vi "GUI_148_AmplifierCamsV2.vi"() -> ()   [LabVIEW 2013]
uses:
  shared programs/GUI_Template/GUI_master/tcp_new_data_event.ctl
  shared programs/GUI_Template/GUI_master/tcp new data cluster.ctl
  <userlib>/_OpenG.lib/array/array.llb/Filter 1D Array with Scalar (String)__ogtk.vi
panel:
  in  "TargetSize.Y::7":dbl=45.0 caption="y" min=2.0 max=3000.0 format="%#_6f"
  in  "TargetSize.X::7":dbl=47.0 caption="x" min=2.0 max=3000.0 format="%#_6f"
  in  "TargetSize.Y::6":dbl=45.0 caption="y" min=2.0 max=3000.0 format="%#_6f"
  in  "TargetSize.X::6":dbl=47.0 caption="x" min=2.0 max=3000.0 format="%#_6f"
  in  "TargetSize.Y::5":dbl=45.0 caption="y" min=2.0 max=3000.0 format="%#_6f"
  in  "TargetSize.X::5":dbl=47.0 caption="x" min=2.0 max=3000.0 format="%#_6f"
  in  "TargetSize.Y::4":dbl=45.0 caption="y" min=2.0 max=3000.0 format="%#_6f"
  in  "TargetSize.X::4":dbl=47.0 caption="x" min=2.0 max=3000.0 format="%#_6f"
  in  "TargetSize.Y::3":dbl=163.0 caption="y" min=2.0 max=3000.0 format="%#_6f"
  in  "TargetSize.X::3":dbl=152.0 caption="x" min=2.0 max=3000.0 format="%#_6f"
  in  "TargetSize.Y::2":dbl=74.0 caption="y" min=2.0 max=3000.0 format="%#_6f"
  in  "TargetSize.X::2":dbl=75.0 caption="x" min=2.0 max=3000.0 format="%#_6f"
  in  "active cams":string
  out "CCDs":string[](array[string])
  out "Cameras":T1
  in  "Target.Y::7":dbl=45.0 caption="y" min=0.0 max=2000.0 format="%#_6f"
  in  "Target.X::7":dbl=47.0 caption="x" min=0.0 max=2000.0 format="%#_6f"
  in  "Target.Y::6":dbl=45.0 caption="y" min=0.0 max=2000.0 format="%#_6f"
  in  "Target.X::6":dbl=47.0 caption="x" min=0.0 max=2000.0 format="%#_6f"
  in  "Target.Y::5":dbl=45.0 caption="y" min=0.0 max=2000.0 format="%#_6f"
  in  "Target.X::5":dbl=47.0 caption="x" min=0.0 max=2000.0 format="%#_6f"
  in  "Target.Y::4":dbl=45.0 caption="y" min=0.0 max=2000.0 format="%#_6f"
  in  "Target.X::4":dbl=47.0 caption="x" min=0.0 max=2000.0 format="%#_6f"
  in  "Target.Y::3":dbl=163.0 caption="y" min=0.0 max=2000.0 format="%#_6f"
  in  "Target.X::3":dbl=152.0 caption="x" min=0.0 max=2000.0 format="%#_6f"
  in  "Target.Y::2":dbl=74.0 caption="y" min=0.0 max=2000.0 format="%#_6f"
  in  "Target.X::2":dbl=75.0 caption="x" min=0.0 max=2000.0 format="%#_6f"
  out "error out":errorcluster
  out "image::7":T2(plugin-control) caption="U_Amp3GaiaBay"
  in  "triggerdelay::7":dbl=0.001 caption="triggerdelay" min=0.0 max=50000.0 format="%_4p"
  in  "triggerdelay::6":dbl=0.001 caption="triggerdelay" min=20.0 max=50000.0 format="%_4p"
  in  "triggerdelay::5":dbl=0.001 caption="triggerdelay" min=10.0 max=50000.0 format="%_4p"
  in  "triggerdelay::4":dbl=0.001 caption="triggerdelay" min=0.0 max=50000.0 format="%_4p"
  in  "triggerdelay::3":dbl=0.001 caption="triggerdelay" min=20.0 max=50000.0 format="%_4p"
  in  "triggerdelay::2":dbl=0.001 caption="triggerdelay" min=0.0 max=50000.0 format="%_4p"
  in  "trigger::7":bool caption="Trigger"
  in  "centroidy::7":dbl=0.001 caption="centroid y" min=0.0 max=0.0 format="%_4f"
  in  "centroidx::7":dbl=0.001 caption="centroid x" min=0.0 max=0.0 format="%_4f"
  in  "exposure::7":dbl=0.001 caption="exposure" min=0.0001 max=1.0 format="%_4p"
  in  "GUIdevice 7":string="U_GAIACam"
  in  "trigger::6":bool caption="Trigger"
  in  "centroidy::6":dbl=0.001 caption="centroid y" min=0.0 max=0.0 format="%_4f"
  in  "centroidx::6":dbl=0.001 caption="centroid x" min=0.0 max=0.0 format="%_4f"
  in  "exposure::6":dbl=0.001 caption="exposure" min=0.0001 max=1.0 format="%_4p"
  out "image::6":T2(plugin-control) caption="U_Amp3GaiaBay"
  in  "GUIdevice 6":string="U_Amp3GaiaBay"
  in  "trigger::5":bool caption="Trigger"
  in  "centroidy::5":dbl=0.001 caption="centroid y" min=0.0 max=0.0 format="%_4f"
  in  "centroidx::5":dbl=0.001 caption="centroid x" min=0.0 max=0.0 format="%_4f"
  in  "exposure::5":dbl=0.001 caption="exposure" min=0.0001 max=1.0 format="%_4p"
  out "image::5":T2(plugin-control) caption="U_Amp2GaiaBay"
  in  "GUIdevice 5":string="U_Amp2GaiaBay"
  in  "trigger::4":bool caption="Trigger"
  in  "centroidy::4":dbl=0.001 caption="centroid y" min=0.0 max=0.0 format="%_4f"
  in  "centroidx::4":dbl=0.001 caption="centroid x" min=0.0 max=0.0 format="%_4f"
  in  "exposure::4":dbl=0.001 caption="exposure" min=1e-06 max=1.0 format="%_4p"
  out "image::4":T2(plugin-control) caption="U_IRMobileImager"
  in  "GUIdevice 4":string="U_IRMobileImager"
  in  "trigger::3":bool caption="Trigger"
  in  "centroidy::3":dbl=0.001 caption="centroid y" min=0.0 max=0.0 format="%_4f"
  in  "centroidx::3":dbl=0.001 caption="centroid x" min=0.0 max=0.0 format="%_4f"
  in  "exposure::3":dbl=0.001 caption="exposure" min=0.0001 max=1.0 format="%_4p"
  out "image::3":T2(plugin-control) caption="Amp3_IR_Input"
  in  "GUIdevice 3":string="U_Amp3_IR_Input"
  in  "trigger::2":bool caption="Trigger"
  in  "centroidy::2":dbl=0.001 caption="centroid y" min=0.0 max=0.0 format="%_4f"
  in  "centroidx::2":dbl=0.001 caption="centroid x" min=0.0 max=0.0 format="%_4f"
  in  "exposure::2":dbl=0.001 caption="exposure" min=0.0001 max=1.0 format="%_4p"
  out "image::2":T2(plugin-control) caption="Amp2_IR_input"
  in  "GUIdevice 2":string="U_Amp2_IR_input"
  out "tcp data event":T3
  in  "Refresh Button":bool caption="Update Crosshairs"
  in  "Select device":string(combo)="FrogHPD"
  in  "stop":bool
  in  "GUIdevice 1":string="HPD_CCD"
  # "XHair location"
  # "XHair size"
  # "XHair location"
  # "XHair size"
  # "XHair location"
  # "XHair size"
  # "XHair location"
  # "XHair size"
  # "XHair location"
  # "XHair size"
  # "XHair location"
  # "XHair size"
  # "XHair location"
  # "XHair size"
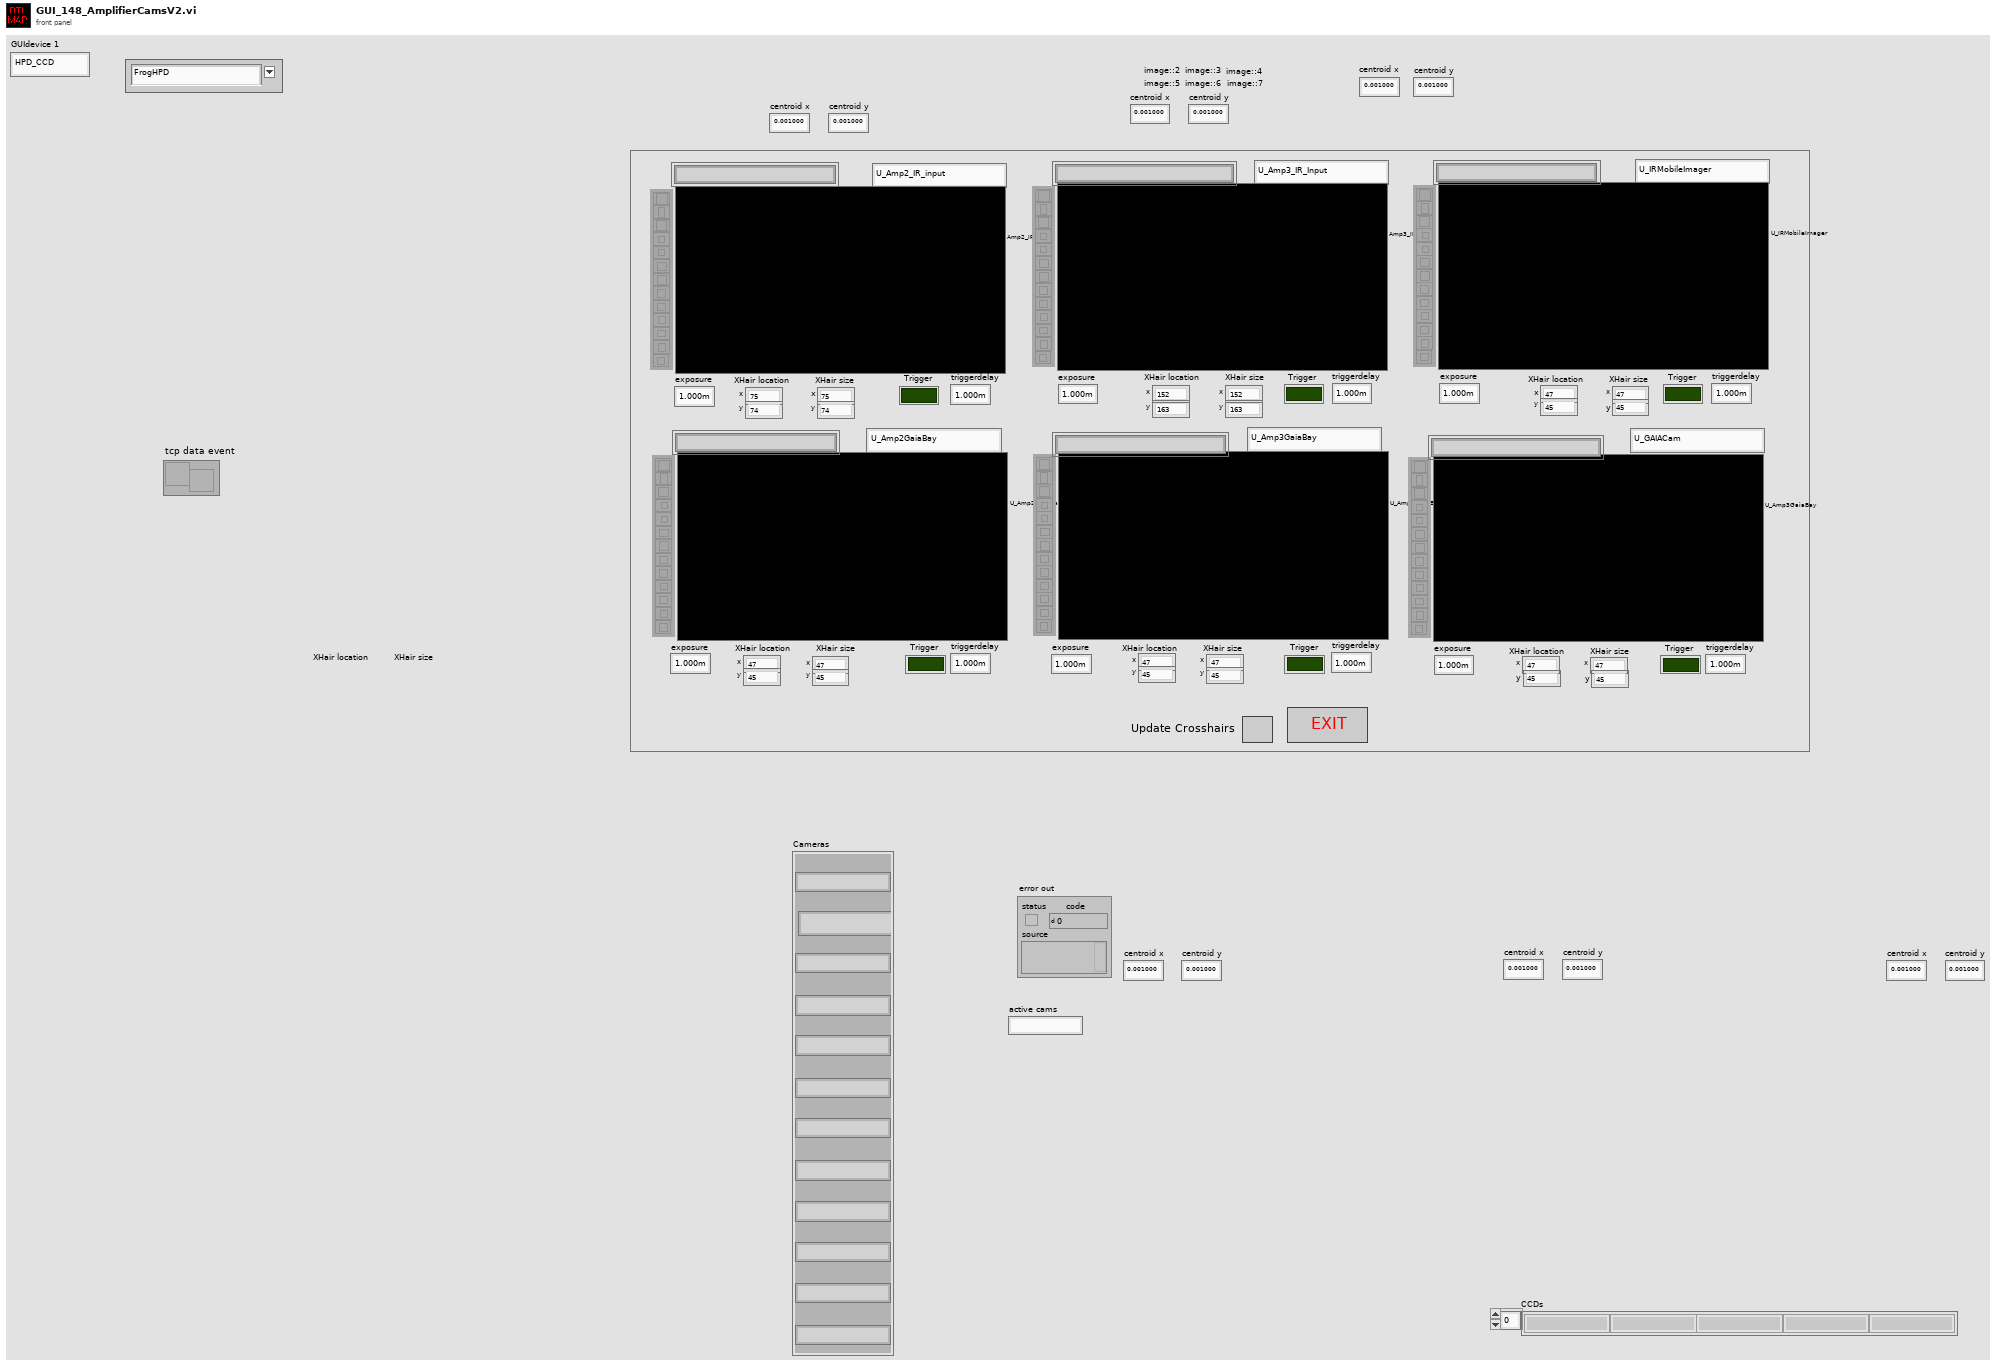
[diagram p1: front panel]
types:
  T1 = cluster{"[0]":string, "[1]":string, "[2]":string, "[3]":string, "[4]":string, "[5]":string, "[6]":string, "[7]":string, "[8]":string, "[8] 2":string, "[8] 3":string, "[8] 4":string}
  T2 = typedef "IMAQ Image.ctl" = refnum<image>
  T3 = typedef "tcp_new_data_event.ctl" = refnum<user-event>
  T4 = typedef "Image Type" = u32
  T5 = cluster{"TargetSize.X::2":refnum<vi>, "TargetSize.Y::2":refnum<vi>}
  T6 = cluster{"TargetSize.X::3":refnum<vi>, "TargetSize.Y::3":refnum<vi>}
  T7 = cluster{"TargetSize.X::4":refnum<vi>, "TargetSize.Y::4":refnum<vi>}
  T8 = cluster{"TargetSize.X::5":refnum<vi>, "TargetSize.Y::5":refnum<vi>}
  T9 = cluster{"TargetSize.X::6":refnum<vi>, "TargetSize.Y::6":refnum<vi>}
  T10 = cluster{"TargetSize.X::7":refnum<vi>, "TargetSize.Y::7":refnum<vi>}
  T11 = cluster{"Target.X::2":refnum<vi>, "Target.Y::2":refnum<vi>}
  T12 = cluster{"Target.X::3":refnum<vi>, "Target.Y::3":refnum<vi>}
  T13 = cluster{"Target.X::4":refnum<vi>, "Target.Y::4":refnum<vi>}
  T14 = cluster{"Target.X::5":refnum<vi>, "Target.Y::5":refnum<vi>}
  T15 = cluster{"Target.X::6":refnum<vi>, "Target.Y::6":refnum<vi>}
  T16 = cluster{"Target.X::7":refnum<vi>, "Target.Y::7":refnum<vi>}
  T17 = cluster{"[0]":string, "[1]":string, "[2]":string, "[3]":string, "[4]":string, "[5]":string, "[6]":string, "[7]":string, "[8]":string, "[9]":string, "[10]":string, "[11]":string}
  T18 = cluster{"TargetSize.X::7":refnum<vi>, "TargetSize.Y::7":refnum<vi>}[]
  T19 = cluster{"Target.X::7":refnum<vi>, "Target.Y::7":refnum<vi>}[]
  T20 = cluster{"Left":i32, "Top":i32, "Right":i32, "Bottom":i32}
  T21 = enum32{"invalid app kind", "Development System", "Run Time System", "Student Edition", "Embedded LabVIEW", "Evaluation", "Custom"}
  T22 = typedef "tcp new data cluster.ctl" = cluster{"EventEnum":enum16{"new data", "connection status update"}, "Device name":string}
  T23 = enum32{"Invalid", "Standard", "Closed", "Hidden", "Minimized", "Maximized"}
  T24 = cluster{"Core":cluster{"Current VI Reference":refnum<vi>, "Close Panel on Exit?":bool}, "Your Boolean data":bool, "active cams":string, "SuperGUI":cluster{"STOP queue":refnum<queue>, "SuperGUI ref":refnum<vi>}}
  T25 = cluster{"STOP queue":refnum<queue>, "SuperGUI ref":refnum<vi>}
  T26 = cluster{"Current VI Reference":refnum<vi>, "Close Panel on Exit?":bool}
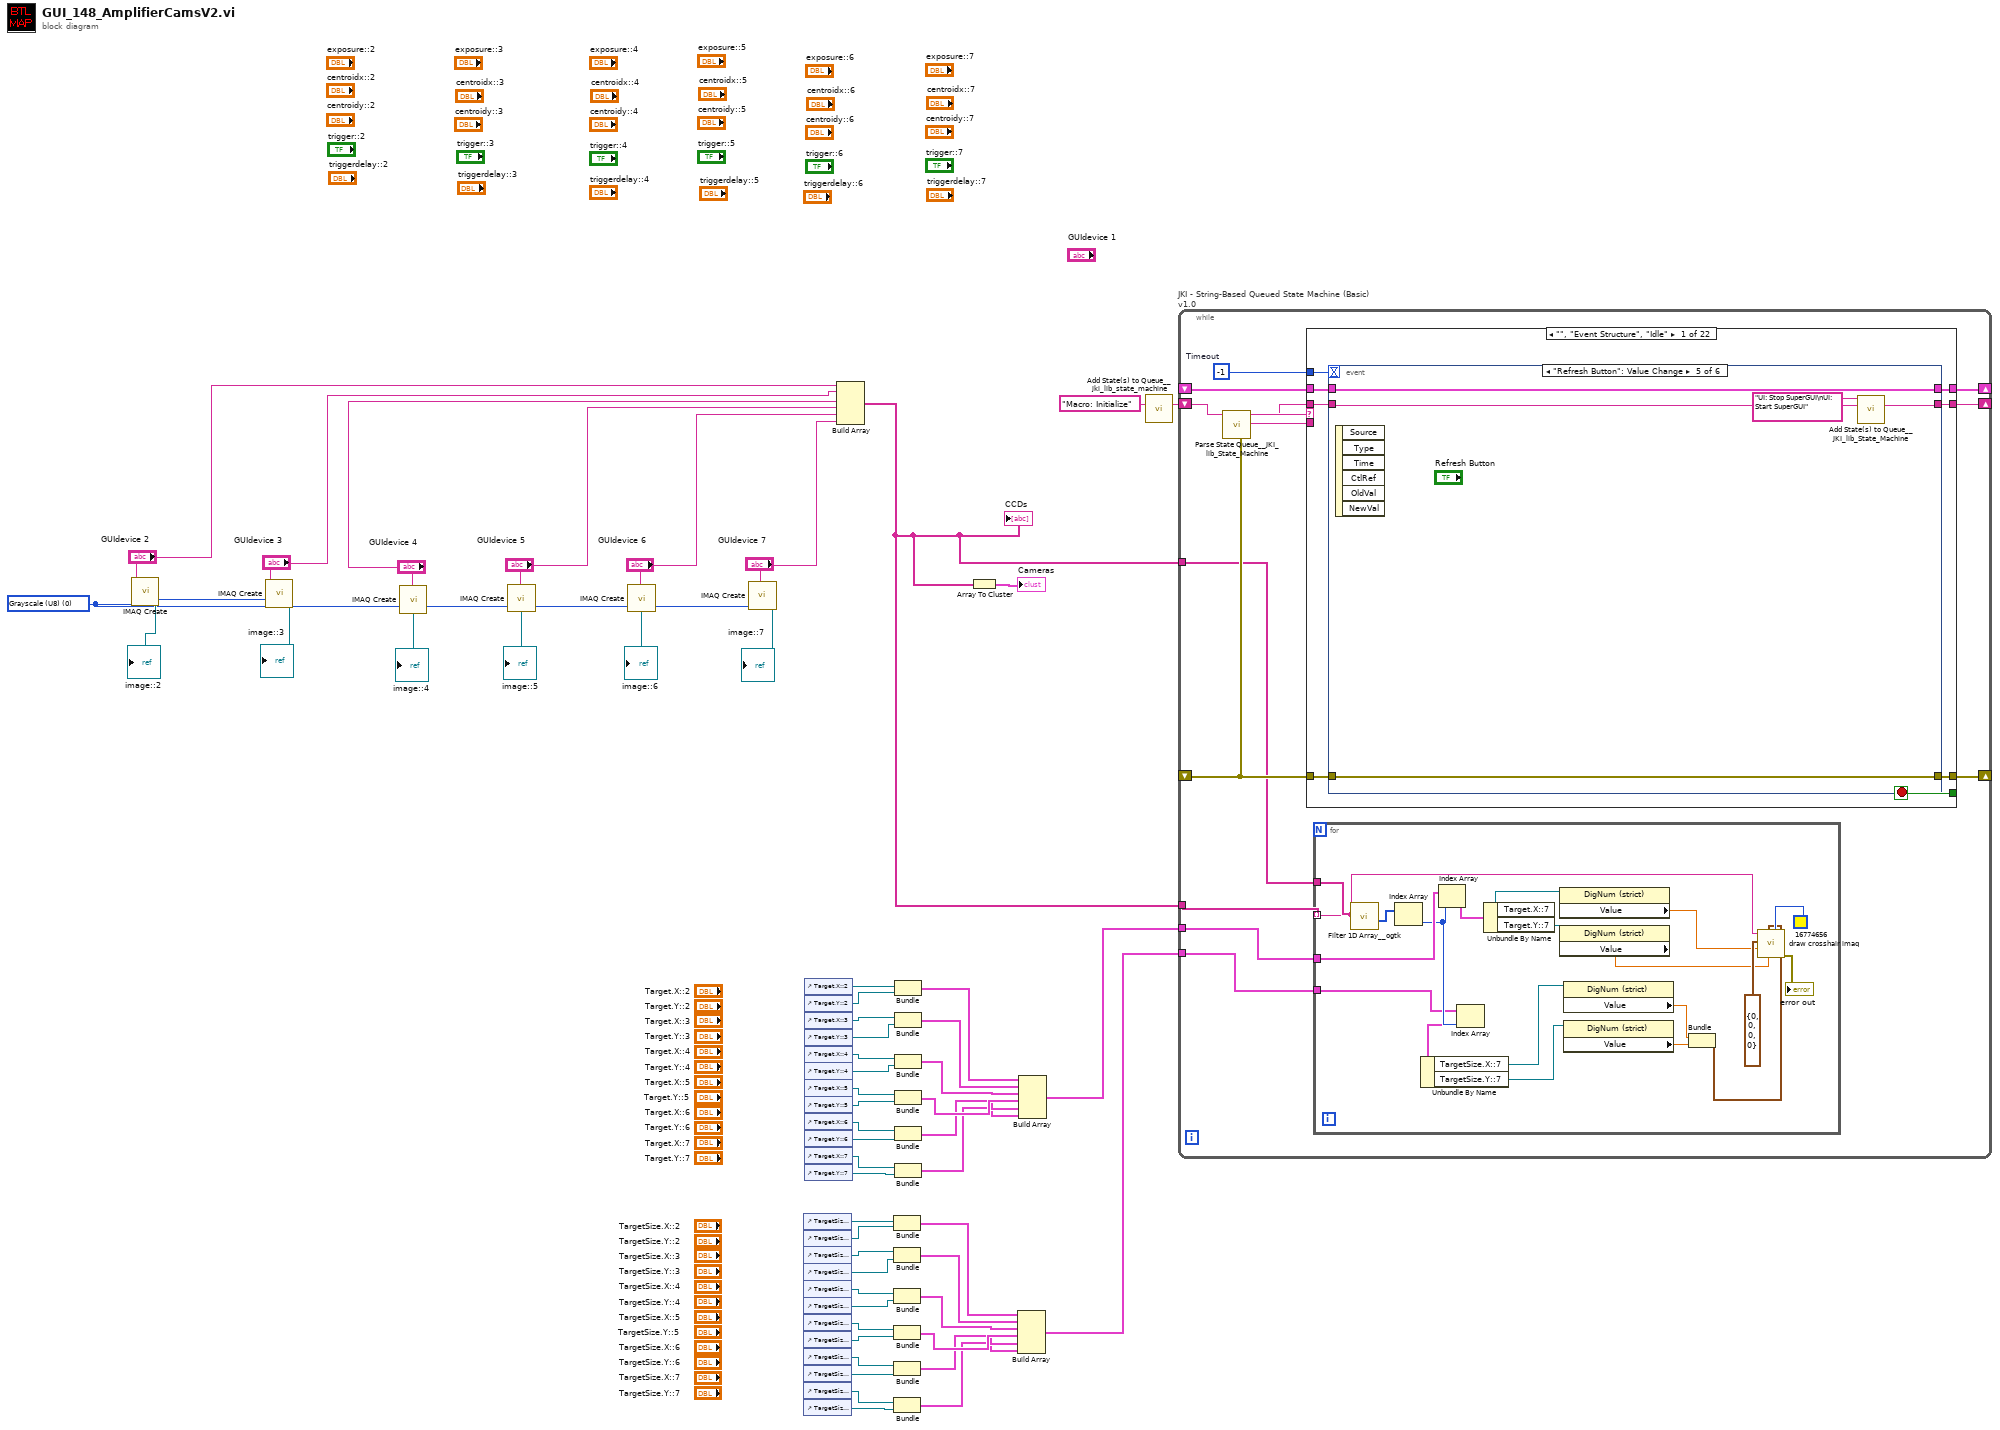
[diagram p0: block diagram]
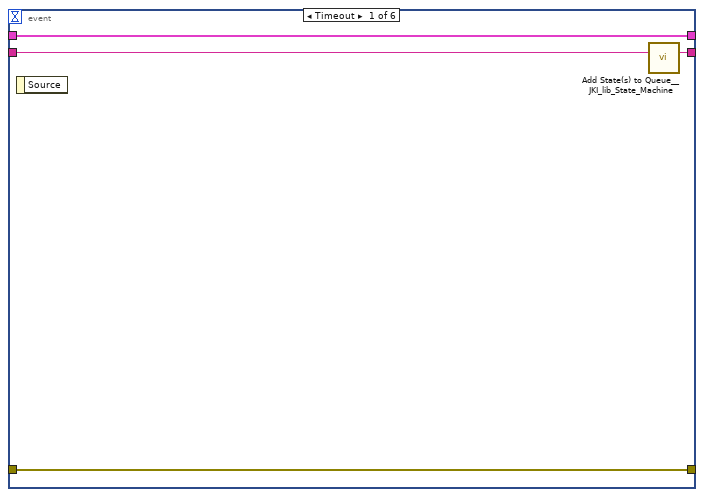
[diagram p2: hidden frame]
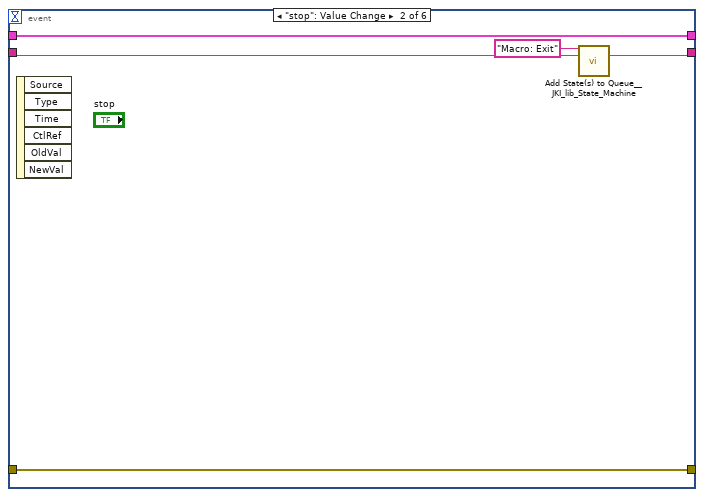
[diagram p3: hidden frame]
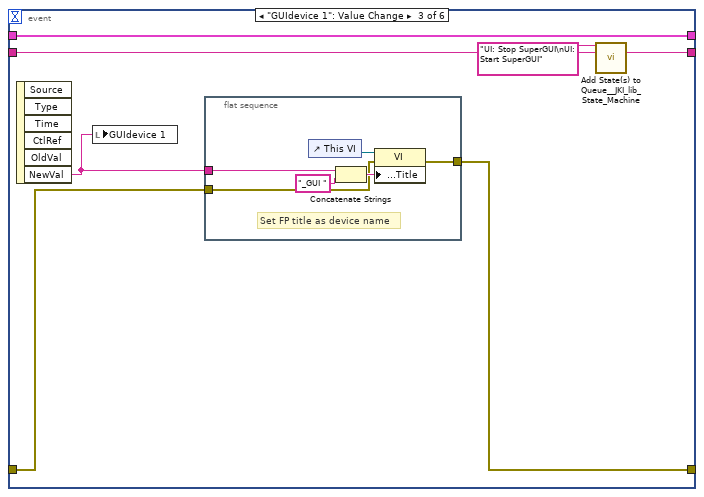
[diagram p4: hidden frame]
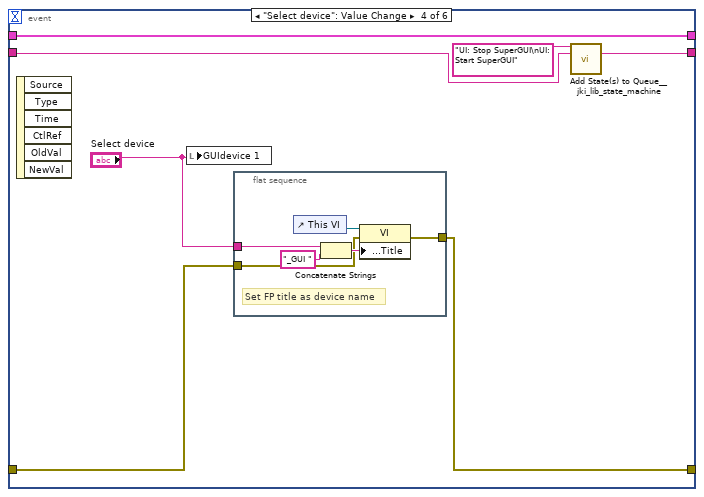
[diagram p5: hidden frame]
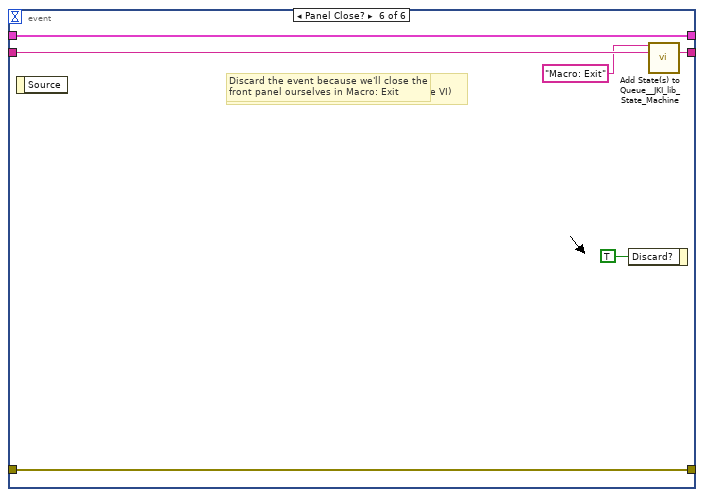
[diagram p6: hidden frame]
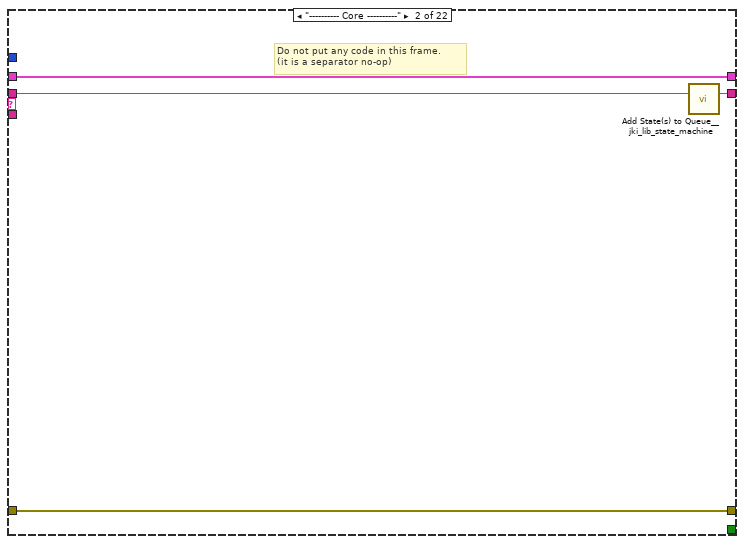
[diagram p7: hidden frame]
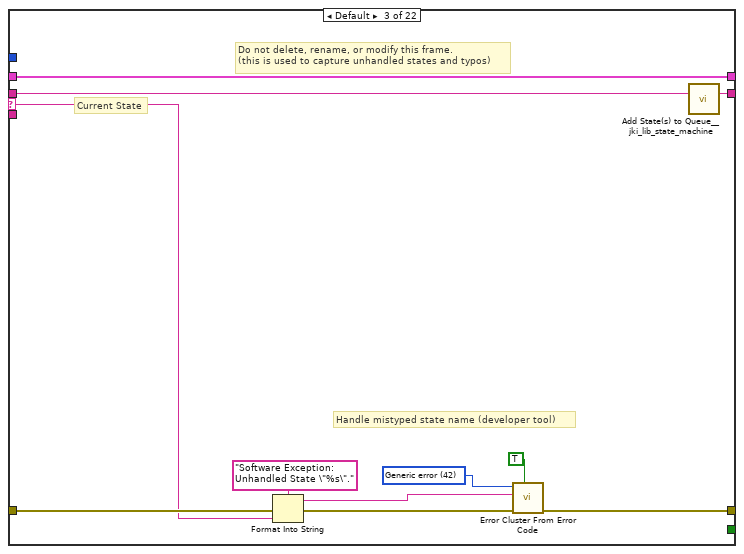
[diagram p8: hidden frame]
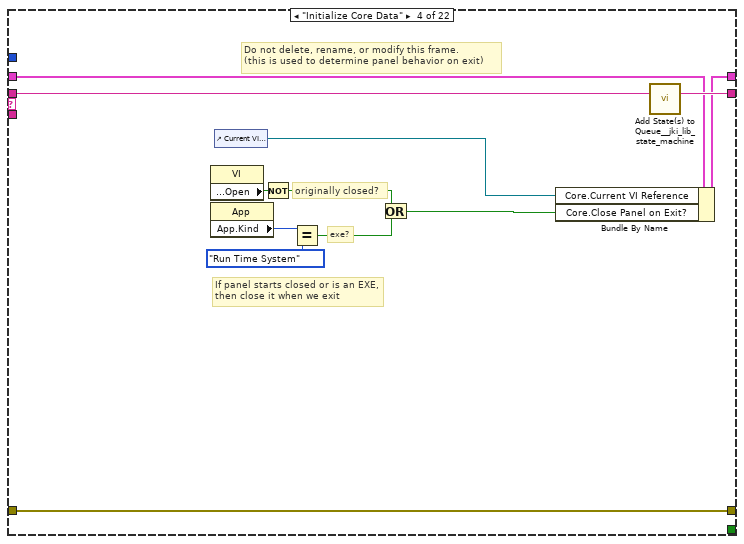
[diagram p9: hidden frame]
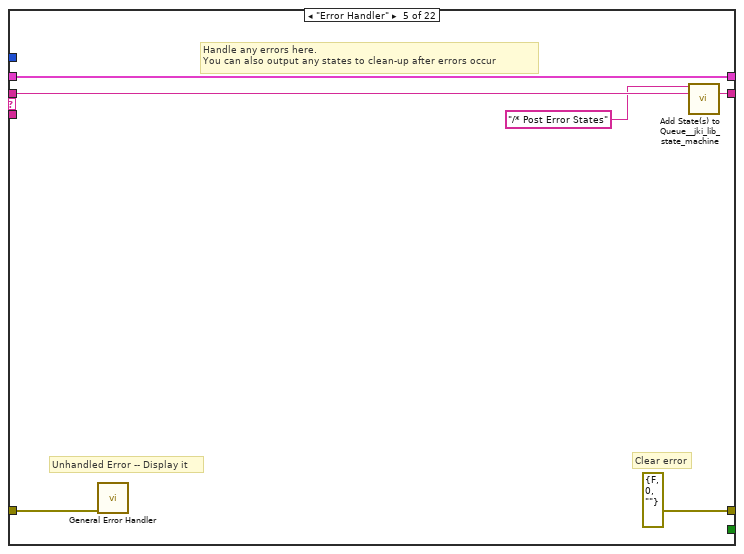
[diagram p10: hidden frame]
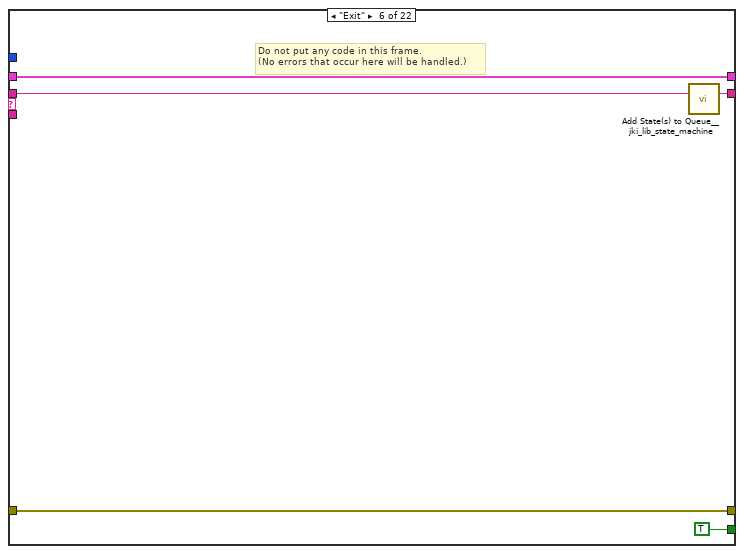
[diagram p11: hidden frame]
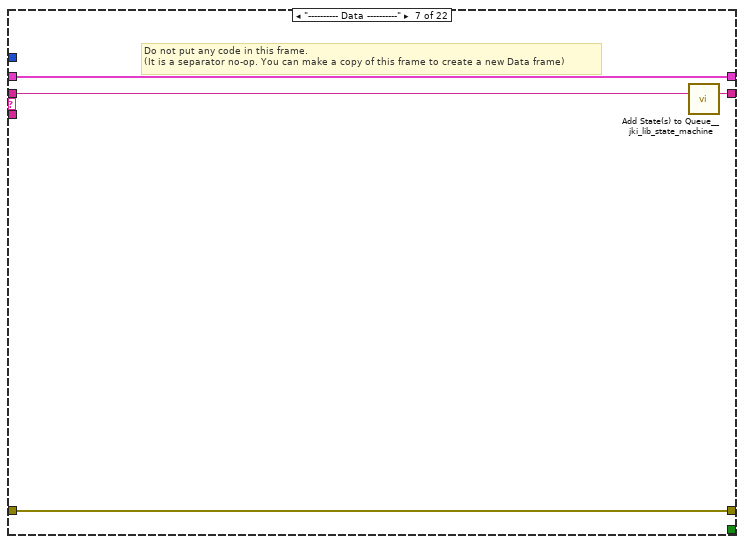
[diagram p12: hidden frame]
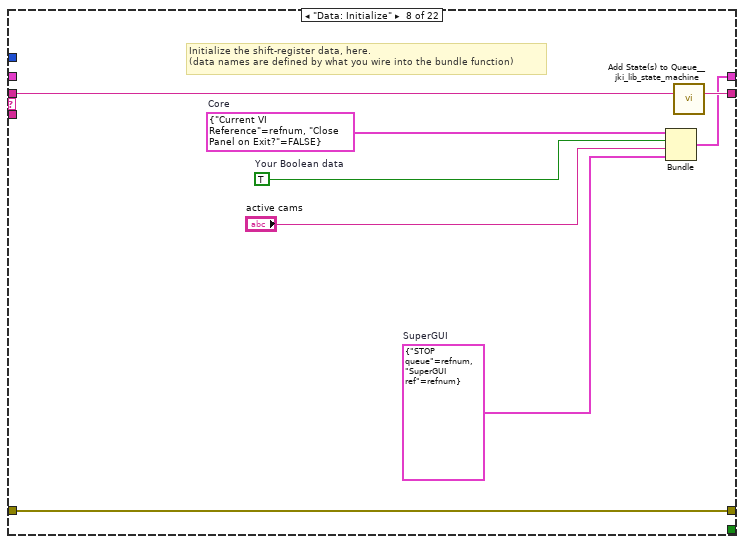
[diagram p13: hidden frame]
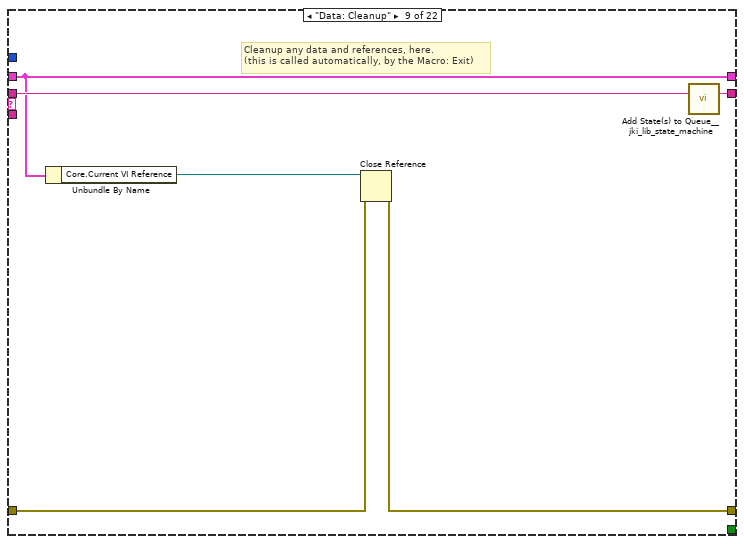
[diagram p14: hidden frame]
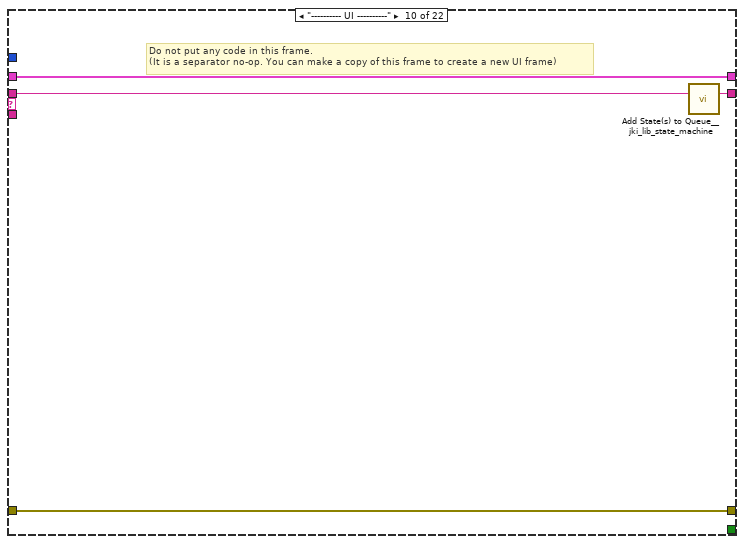
[diagram p15: hidden frame]
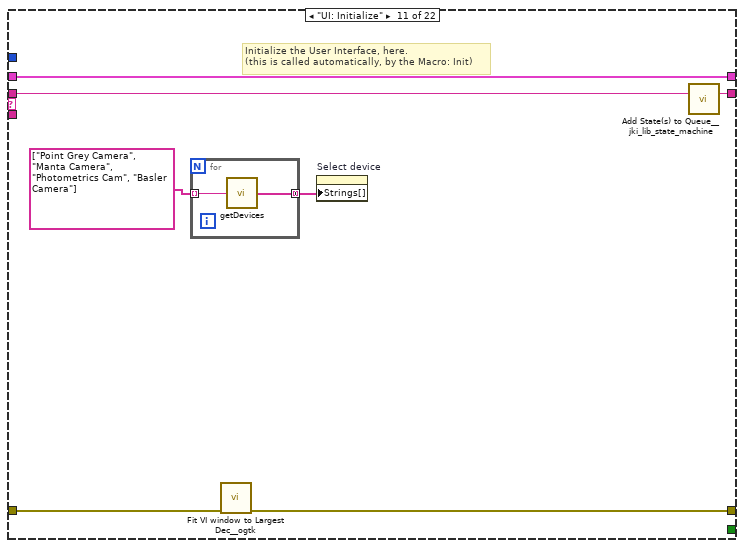
[diagram p16: hidden frame]
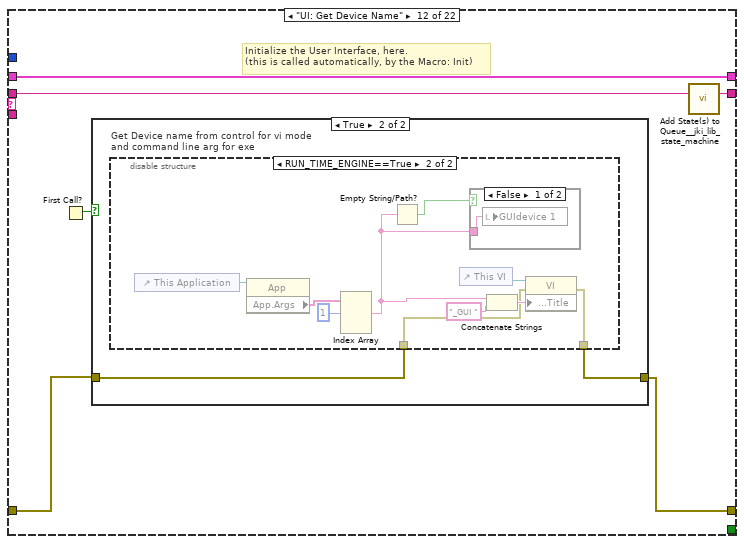
[diagram p17: hidden frame]
diagram:
  w48 = T4 0 items=["Grayscale (U8)", "Grayscale (I16)", "Grayscale (SGL)", "Complex (CSG)", "RGB (U32)", "HSL (U32)", "RGB (U64)", "Grayscale (U16)"] ("Image Type")
  n1 = call "IMAQ Create"("Image Name"="GUIdevice 2", "Image Type"=w48) -> ("New Image"=→"image::2":T2)  [unwired: 3 in, 1 out]
  n2 = call "IMAQ Create"("Image Name"="GUIdevice 3", "Image Type"=w48) -> ("New Image"=→"image::3":T2)  [unwired: 3 in, 1 out]
  n3 = call "IMAQ Create"("Image Name"="GUIdevice 4", "Image Type"=w48) -> ("New Image"=→"image::4":T2)  [unwired: 3 in, 1 out]
  n4 = call "IMAQ Create"("Image Name"="GUIdevice 5", "Image Type"=w48) -> ("New Image"=→"image::5":T2)  [unwired: 3 in, 1 out]
  n5 = call "IMAQ Create"("Image Name"="GUIdevice 6", "Image Type"=w48) -> ("New Image"=→"image::6":T2)  [unwired: 3 in, 1 out]
  n6 = call "IMAQ Create"("Image Name"="GUIdevice 7", "Image Type"=w48) -> ("New Image"=→"image::7":T2)  [unwired: 3 in, 1 out]
  n7 = control-ref of="TargetSize.X::2"() -> (w19:refnum<vi>)
  n8 = control-ref of="TargetSize.Y::2"() -> (w18:refnum<vi>)
  n9 = control-ref of="TargetSize.X::3"() -> (w17:refnum<vi>)
  n10 = control-ref of="TargetSize.Y::3"() -> (w16:refnum<vi>)
  n11 = control-ref of="TargetSize.X::4"() -> (w15:refnum<vi>)
  n12 = control-ref of="TargetSize.Y::4"() -> (w14:refnum<vi>)
  n13 = control-ref of="TargetSize.X::5"() -> (w13:refnum<vi>)
  n14 = control-ref of="TargetSize.Y::5"() -> (w12:refnum<vi>)
  n15 = control-ref of="TargetSize.X::6"() -> (w11:refnum<vi>)
  n16 = control-ref of="TargetSize.Y::6"() -> (w10:refnum<vi>)
  n17 = control-ref of="TargetSize.X::7"() -> (w9:refnum<vi>)
  n18 = control-ref of="TargetSize.Y::7"() -> (w8:refnum<vi>)
  n19 = control-ref of="Target.X::2"() -> (w46:refnum<vi>)
  n20 = control-ref of="Target.Y::2"() -> (w45:refnum<vi>)
  n21 = control-ref of="Target.X::3"() -> (w44:refnum<vi>)
  n22 = control-ref of="Target.Y::3"() -> (w43:refnum<vi>)
  n23 = control-ref of="Target.X::4"() -> (w42:refnum<vi>)
  n24 = control-ref of="Target.Y::4"() -> (w41:refnum<vi>)
  n25 = control-ref of="Target.X::5"() -> (w40:refnum<vi>)
  n26 = control-ref of="Target.Y::5"() -> (w39:refnum<vi>)
  n27 = control-ref of="Target.X::6"() -> (w38:refnum<vi>)
  n28 = control-ref of="Target.Y::6"() -> (w37:refnum<vi>)
  n29 = control-ref of="Target.X::7"() -> (w36:refnum<vi>)
  n30 = control-ref of="Target.Y::7"() -> (w35:refnum<vi>)
  n31 = Build Array("GUIdevice 2", "GUIdevice 3", "GUIdevice 4", "GUIdevice 5", "GUIdevice 6", "GUIdevice 7") -> (w20:string[])
  "CCDs" <- w20
  n32 = Bundle("TargetSize.X::2"=w19, "TargetSize.Y::2"=w18) -> (w7:T5)  [unwired: 1 in]
  n33 = Bundle("TargetSize.X::3"=w17, "TargetSize.Y::3"=w16) -> (w6:T6)  [unwired: 1 in]
  n34 = Bundle("TargetSize.X::4"=w15, "TargetSize.Y::4"=w14) -> (w2:T7)  [unwired: 1 in]
  n35 = Bundle("TargetSize.X::5"=w13, "TargetSize.Y::5"=w12) -> (w5:T8)  [unwired: 1 in]
  n36 = Bundle("TargetSize.X::6"=w11, "TargetSize.Y::6"=w10) -> (w4:T9)  [unwired: 1 in]
  n37 = Bundle("TargetSize.X::7"=w9, "TargetSize.Y::7"=w8) -> (w3:T10)  [unwired: 1 in]
  n38 = Bundle("Target.X::2"=w46, "Target.Y::2"=w45) -> (w34:T11)  [unwired: 1 in]
  n39 = Bundle("Target.X::3"=w44, "Target.Y::3"=w43) -> (w33:T12)  [unwired: 1 in]
  n40 = Bundle("Target.X::4"=w42, "Target.Y::4"=w41) -> (w29:T13)  [unwired: 1 in]
  n41 = Bundle("Target.X::5"=w40, "Target.Y::5"=w39) -> (w32:T14)  [unwired: 1 in]
  n42 = Bundle("Target.X::6"=w38, "Target.Y::6"=w37) -> (w31:T15)  [unwired: 1 in]
  n43 = Bundle("Target.X::7"=w36, "Target.Y::7"=w35) -> (w30:T16)  [unwired: 1 in]
  n44 = Array To Cluster(array=w20) -> (cluster=→"Cameras":T17)
  n45 = Build Array(w7, w6, w2, w5, w4, w3) -> (w1:T18)
  n46 = Build Array(w34, w33, w29, w32, w31, w30) -> (w28:T19)
  n47 = call <vilib>:"Add State(s) to Queue__jki_lib_state_machine.vi"("State(s) in (\"\")"="Macro: Initialize") -> ("States Out"=w55:string)  [unwired: 14 in]
  n48 = while "JKI - String-Based Queued State Machine (Basic) v1.0" {
    shift-right: [w63] -> _
    shift-left: _ -> [w58]
    shift-right: [w66] -> _
    shift-left: _ -> [w61]
    shift-right: [w65] -> _
    shift-left: w55 -> [w67]
    tunnel: w28 -> [w60]
    tunnel: w20 -> [w59]
    tunnel: w20 -> [w57]
    tunnel: w1 -> [w56]
    stop <- w64 stop-if-true
    w62 = -1  # Timeout
    n49 = call <vilib>:"Parse State Queue__JKI_lib_State_Machine.vi"("State Queue"=w67, "Error In (no error)"=w61) -> ("Remaining States"=w69:string, "Current State"=w70:string, "Arguments"=w68:string)  [unwired: 11 in]
    n50 = case shown="\"\", \"Event Structure\", \"Idle\"" w70 {
      selector: w70 -> [_ _ w148 _ _ _ _ _ _ _ _ _ _ _ _ _ _ _ _ _ _ _]
      tunnel: w69 -> [w97 w147 w152 w170 w176 w181 w185 w193 w199 w203 w210 w218 w253 w261 w267 w278 w304 w309 w319 w323 w327 w331]
      tunnel: w68 -> [_ _ _ _ _ _ _ _ _ _ _ _ _ _ w262 w272 _ _ _ _ _ _]
      tunnel: w58 -> [w95 w144 w150 w161 w173 w179 w182 _ w194 w200 w208 w216 w244 w256 w265 w274 w301 w306 w316 w320 w324 w328]
      tunnel: [w94 w145 w154 w167 errorcluster {"status"=FALSE, "code"=0, "source"=""} ("error out") w178 w183 w190 w195 w201 w206 w213 w237 w254 w263 w275 w302 w307 w317 w321 w325 w329] -> w66
      tunnel: w61 -> [w93 w145 w153 w167 w172 w178 w183 w190 w196 w201 w207 w214 w238 w255 w264 w276 w302 w307 w317 w321 w325 w329]
      tunnel: [w96 w146 w151 w169 w175 w180 w184 w192 w198 w202 w209 w217 w252 w260 w266 w277 w303 w308 w318 w322 w326 w330] -> w65
      tunnel: [_ _ _ _ _ TRUE _ _ _ _ _ _ _ _ _ _ _ _ _ _ _ _] -> w64
      tunnel: [w92 w144 w150 w168 w173 w179 w182 w191 w194 w200 w208 w216 w243 w256 w265 w274 w301 w306 w316 w320 w324 w328] -> w63
      tunnel: w62 -> [w91 _ _ _ _ _ _ _ _ _ _ _ _ _ _ _ _ _ _ _ _ _]
      frame "", "Event Structure", "Idle" {
        n51 = event shown="[4] \"Refresh Button\": Value Change" {
          selector: _ -> [_ _ _ _ _ _]
          dyn-events: _ -> [_ _ _ _ _ _]
          timeout: w91 -> [_ _ _ _ _ _]
          tunnel: w97 -> [w101 w104 w110 w122 w135 w143]
          tunnel: [w100 w103 w109 w121 w134 w142] -> w96
          tunnel: w95 -> [w98 w106 w113 w126 w137 w140]
          tunnel: [w99 w105 w111 w124 w136 w141] -> w94
          tunnel: w93 -> [w99 w105 w112 w125 w136 w141]
          tunnel: [w98 w106 w113 w126 w137 w140] -> w92
          event Timeout {
            n52 = event-data() -> ()  [unwired: 1 in, 1 out]
            n53 = call <vilib>:"Add State(s) to Queue__JKI_lib_State_Machine.vi"("State(s) in (\"\")"=w101) -> ("States Out"=w100:string)  [unwired: 14 in]
          }
          event "stop": Value Change {
            n54 = event-data() -> ()  [unwired: 1 in, 6 out]
            n55 = call <vilib>:"Add State(s) to Queue__JKI_lib_State_Machine.vi"("State(s) in Front (\"\")"="Macro: Exit", "State(s) in (\"\")"=w104) -> ("States Out"=w103:string)  [unwired: 13 in]
          }
          event "GUIdevice 1": Value Change {
            n56 = event-data() -> ("NewVal"=w107:string)  [unwired: 1 in, 5 out]
            n57 = local write "GUIdevice 1"(w107) -> ()
            n58 = flat-sequence {
              tunnel: [w116] -> w111
              tunnel: w112 -> [w115]
              tunnel: w107 -> [w114]
              frame #0 {
                # "Set FP title as device name"
                n59 = control-ref of="This VI"() -> (w119:refnum<vi>)
                n60 = Concatenate Strings(w114, "_GUI ") -> (w118:string)
                n61 = property class="VI"(reference=w119, error in=w115, "Front Panel.Title"=w118) -> (error out=w116:errorcluster)  [unwired: 1 out]
              }
            }
            n62 = call <vilib>:"Add State(s) to Queue__JKI_lib_State_Machine.vi"("State(s) in Front (\"\")"="UI: Stop SuperGUI\nUI: Start SuperGUI", "State(s) in (\"\")"=w110) -> ("States Out"=w109:string)  [unwired: 13 in]
          }
          event "Select device": Value Change {
            n63 = event-data() -> ()  [unwired: 1 in, 6 out]
            n64 = local write "GUIdevice 1"("Select device") -> ()
            n65 = flat-sequence {
              tunnel: [w129] -> w124
              tunnel: w125 -> [w128]
              tunnel: "Select device" -> [w127]
              frame #0 {
                # "Set FP title as device name"
                n66 = control-ref of="This VI"() -> (w132:refnum<vi>)
                n67 = Concatenate Strings(w127, "_GUI ") -> (w131:string)
                n68 = property class="VI"(reference=w132, error in=w128, "Front Panel.Title"=w131) -> (error out=w129:errorcluster)  [unwired: 1 out]
              }
            }
            n69 = call <vilib>:"Add State(s) to Queue__jki_lib_state_machine.vi"("State(s) in Front (\"\")"="UI: Stop SuperGUI\nUI: Start SuperGUI", "State(s) in (\"\")"=w122) -> ("States Out"=w121:string)  [unwired: 13 in]
          }
          event "Refresh Button": Value Change {
            n70 = event-data() -> ()  [unwired: 1 in, 6 out]
            n71 = call <vilib>:"Add State(s) to Queue__JKI_lib_State_Machine.vi"("State(s) in Front (\"\")"="UI: Stop SuperGUI\nUI: Start SuperGUI", "State(s) in (\"\")"=w135) -> ("States Out"=w134:string)  [unwired: 13 in]
          }
          event Panel Close? {
            # "Discard the event because we'll close the front panel ourselves in Macro: Exit"
            # "Close Panel button (pressed) Event\n(this executes Macro: Exit to terminate the VI)"
            n72 = event-data() -> ()  [unwired: 1 in, 1 out]
            n73 = event-data("Discard?"=TRUE) -> ()  [unwired: 1 in, 1 out]
            n74 = call <vilib>:"Add State(s) to Queue__JKI_lib_State_Machine.vi"("State(s) in Front (\"\")"="Macro: Exit", "State(s) in (\"\")"=w143) -> ("States Out"=w142:string)  [unwired: 13 in]
          }
        }
      }
      frame "---------- Core ----------" {
        # "Do not put any code in this frame.\n(it is a separator no-op)"
        n75 = call <vilib>:"Add State(s) to Queue__jki_lib_state_machine.vi"("State(s) in (\"\")"=w147) -> ("States Out"=w146:string)  [unwired: 14 in]
      }
      frame Default {
        w157 = 42 items=["No error", "Argument error", "Memory is full", "Out of zone", "End of file", "File already open", "Generic file I/O error", "File not found", "File permission error", "Disk is full", "Duplicate path", "Too many files open", "System feature not enabled", "Resource file not found", "Cannot add resource", "Resource not found", "Image not found", "Image memory error", "Pen does not exist", "Config type invalid", "Config token not found", "Config parse error", "Config memory error", "Bad external code format", "Bad external code offset", "External code not present", "Null window", "Destroy window error", "Null menu", "Print aborted", "Bad print record", "Print driver error", "Windows error during printing", "Memory error during printing", "Print dialog error", "Generic print error", "Invalid device refnum", "Device not found", "Device parameter error", "Device unit error", "Cannot open device", "Device call aborted", "Generic error", "Cancelled by user", "Object ID too low", "Object ID too high", "Object not in heap", "Unknown heap", "Unknown object (invalid DefProc)", "Unknown object (DefProc not in table)", "Message out of range", "Invalid (null) method", "Unknown message", "Manager call not supported", "Bad address", "Network operation in progress", "Network operation timed out", "Connection is busy", "Network attribute not supported", "Network error", "Address in use", "System out of memory", "Connection aborted", "Connection refused", "Not connected", "Already connected", "Connection closed", "Initialization error (interapplication manager)", "Bad occurrence", "Wait on unbound occurrence handler", "Occurrence queue overflow", "Datalog type conflict", "Unused", "Unrecognized type (interapplication manager)", "Memory corrupt", "Failed to make temporary DLL", "Old CIN version", "Drag socket not found", "Failed to load drop-object", "Failed to register OLE object", "Failed to release OLE object", "Format specifier type mismatch", "Unknown format specifier", "Too few format specifiers", "Too many format specifiers", "Scan failed", "Newer CIN version", "Error converting to variant", "Runtime menu error", "Password tampered", "Variant attribute not found", "Incompatible variant data type", "Event data is not available", "Event Store is not present", "Occurrence is not found", "Event Queue is not created", "Event info is not available", "Refnum passed is NULL", "Error retrieving Class GUID", "Error retrieving CoClass GUID", "Error retrieving TypeLib GUID.", "Bad built application magic bytes.", "Specific driver is different from the specific driver associated with the Logical Name.", "There is no session opened to the class driver.", "Max Error", "MAX - Error with config objects", "MAX - Error loading configuration", "MAX - Group not supported"]
        # "Current State"
        # "Do not delete, rename, or modify this frame.\n(this is used to capture unhandled states and typos)"
        # "Handle mistyped state name (developer tool)"
        n76 = Format Into String(format string="Software Exception: Unhandled State \"%s\"." ("message"), error in=w153, w148) -> (resulting string=w156:string, error out=w155:errorcluster)  [unwired: 1 in]
        n77 = call <vilib>:"Error Cluster From Error Code.vi"("show call chain? (False)"=TRUE, "error in (no error)"=w155, "error message (\"\")"=w156, "error code (0)"=w157) -> ("error out"=w154:errorcluster)  [unwired: 5 in]
        n78 = call <vilib>:"Add State(s) to Queue__jki_lib_state_machine.vi"("State(s) in (\"\")"=w152) -> ("States Out"=w151:string)  [unwired: 14 in]
      }
      frame "Initialize Core Data" {
        # "Do not delete, rename, or modify this frame.\n(this is used to determine panel behavior on exit)"
        # "originally closed?"
        # "exe?"
        # "If panel starts closed or is an EXE, then close it when we exit"
        n79 = property class="VI"() -> ("Front Panel.Open"=w166:bool)  [unwired: 2 in, 2 out]
        n80 = property class="App"() -> ("App.Kind"=w165:T21)  [unwired: 2 in, 2 out]
        n81 = control-ref of="Current VI Reference"() -> (w159:refnum<vi>)
        n82 = Not(x=w166) -> (.not. x?=w163:bool)
        n83 = Equal?(x=w165, y=T21."Run Time System" ("Application:Kind")) -> (x = y?=w162:bool)
        n84 = Or(x=w163, y=w162) -> (x .or. y?=w160:bool)
        n85 = Bundle By Name(cluster=w161, "Core.Current VI Reference"=w159, "Core.Close Panel on Exit?"=w160) -> (w168:T24)
        n86 = call <vilib>:"Add State(s) to Queue__jki_lib_state_machine.vi"("State(s) in (\"\")"=w170) -> ("States Out"=w169:string)  [unwired: 14 in]
      }
      frame "Error Handler" {
        # "Unhandled Error -- Display it"
        # "Handle any errors here.\nYou can also output any states to clean-up after errors occur"
        # "Clear error"
        n87 = call <vilib>:"General Error Handler.vi"("error in (no error)"=w172) -> ()  [unwired: 10 in, 5 out]
        n88 = call <vilib>:"Add State(s) to Queue__jki_lib_state_machine.vi"("State(s) in Front (\"\")"="/* Post Error States", "State(s) in (\"\")"=w176) -> ("States Out"=w175:string)  [unwired: 13 in]
      }
      frame "Exit" {
        # "Do not put any code in this frame.\n(No errors that occur here will be handled.)"
        n89 = call <vilib>:"Add State(s) to Queue__jki_lib_state_machine.vi"("State(s) in (\"\")"=w181) -> ("States Out"=w180:string)  [unwired: 14 in]
      }
      frame "---------- Data ----------" {
        # "Do not put any code in this frame.\n(It is a separator no-op. You can make a copy of this frame to create a new Data frame)"
        n90 = call <vilib>:"Add State(s) to Queue__jki_lib_state_machine.vi"("State(s) in (\"\")"=w185) -> ("States Out"=w184:string)  [unwired: 14 in]
      }
      frame "Data: Initialize" {
        w186 = T25 {"STOP queue"=refnum, "SuperGUI ref"=refnum}  # SuperGUI
        w187 = T26 {"Current VI Reference"=refnum, "Close Panel on Exit?"=FALSE}  # Core
        w189 = TRUE  # Your Boolean data
        # "Initialize the shift-register data, here.\n(data names are defined by what you wire into the bundle function)"
        n91 = Bundle("Core"=w187, "Your Boolean data"=w189, "active cams"="active cams", "SuperGUI"=w186) -> (w191:T24)  [unwired: 1 in]
        n92 = call <vilib>:"Add State(s) to Queue__jki_lib_state_machine.vi"("State(s) in (\"\")"=w193) -> ("States Out"=w192:string)  [unwired: 14 in]
      }
      frame "Data: Cleanup" {
        # "Cleanup any data and references, here.\n(this is called automatically, by the Macro: Exit)"
        n93 = Unbundle By Name(w194) -> ("Core.Current VI Reference"=w197:refnum<vi>)
        n94 = Close Reference(reference=w197, error in (no error)=w196) -> (error out=w195:errorcluster)
        n95 = call <vilib>:"Add State(s) to Queue__jki_lib_state_machine.vi"("State(s) in (\"\")"=w199) -> ("States Out"=w198:string)  [unwired: 14 in]
      }
      frame "---------- UI ----------" {
        # "Do not put any code in this frame.\n(It is a separator no-op. You can make a copy of this frame to create a new UI frame)"
        n96 = call <vilib>:"Add State(s) to Queue__jki_lib_state_machine.vi"("State(s) in (\"\")"=w203) -> ("States Out"=w202:string)  [unwired: 14 in]
      }
      frame "UI: Initialize" {
        # "Initialize the User Interface, here.\n(this is called automatically, by the Macro: Init)"
        n97 = for {
          tunnel: string[] ["Point Grey Camera", "Manta Camera", "Photometrics Cam", "Basler Camera"] -> [w212] mode=indexing
          tunnel: [w211] -> w204 mode=concatenating
          n98 = call "getDevices.vi"("Device Class"=w212) -> ("All Devices"=w211:string[])
        }
        n99 = call <userlib>:"Fit VI window to Largest Dec__ogtk.vi"("error in (no error)"=w207) -> ("error out"=w206:errorcluster)  [unwired: 5 in, 1 out]
        n100 = property on="Select device" class="CmbBox"("Strings[]"=w204) -> ()  [unwired: 2 in, 2 out]
        n101 = call <vilib>:"Add State(s) to Queue__jki_lib_state_machine.vi"("State(s) in (\"\")"=w210) -> ("States Out"=w209:string)  [unwired: 14 in]
      }
      frame "UI: Get Device Name" {
        # "Initialize the User Interface, here.\n(this is called automatically, by the Macro: Init)"
        n102 = First Call?() -> (First Call?: T/F=w215:bool)
        n103 = case shown="True" w215 {
          tunnel: w214 -> [w219 w221]
          tunnel: [w219 w220] -> w213
          frame False {
          }
          frame True {
            n104 = disable-structure "Get Device name from control for vi mode\nand command line arg for exe" shown="RUN_TIME_ENGINE==True" {
              disable-tunnel: w221 -> [w222 w224]
              disable-tunnel: [w222 w223] -> w220
              frame condition #0 (active) {
              }
              frame condition #1 {
                n105 = control-ref of="This Application"() -> (w232:refnum<vi>)
                n106 = property class="App"(reference=w232) -> ("App.Args"=w231:string[])  [unwired: 1 in, 2 out]
                n107 = Index Array(array=w231, index #1=1 ("index")) -> (element #1=w225:string)  [unwired: 2 in, 2 out]
                n108 = Empty String/Path?(string/path=w225) -> (empty?=w229:bool)
                n109 = control-ref of="This VI"() -> (w228:refnum<vi>)
                n110 = case shown="False" w229 {
                  tunnel: w225 -> [w233 _]
                  frame False {
                    n111 = local write "GUIdevice 1"(w233) -> ()
                  }
                  frame True {
                  }
                }
                n112 = Concatenate Strings(w225, "_GUI ") -> (w227:string)
                n113 = property class="VI"(reference=w228, error in=w224, "Front Panel.Title"=w227) -> (error out=w223:errorcluster)  [unwired: 1 out]
              }
            }
          }
        }
        n114 = call <vilib>:"Add State(s) to Queue__jki_lib_state_machine.vi"("State(s) in (\"\")"=w218) -> ("States Out"=w217:string)  [unwired: 14 in]
      }
      frame "UI: Start SuperGUI" {
        # "create stop queue for supergui and its clones"
        # "x100 abort will be dependent on caller VI\nx80 abort will be independent of caller vi, this will abort vi when labview is closed."
        # "Start SuperGUI asynchronous way"
        n115 = vi-ref "GUI_Master_subvi_reentrant_queues.vi"() -> (w236:refnum<vi>)
        n116 = property class="VI"(reference=w236) -> ("Path"=w235:path)  [unwired: 1 in, 2 out]
        n117 = Create User Event(user event datatype=T22 {"EventEnum"=enum."new data", "Device name"="Device name"} ("New Event"), error in=w238) -> (user event=w239:refnum<user-event>, error out=w245:errorcluster)
        "tcp data event" <- w239
        n118 = control-ref of="This Application"() -> (w242:refnum<vi>)
        n119 = control-ref of="This VI"() -> (w241:refnum<vi>)
        n120 = Open VI Reference(type specifier VI Refnum (for type only)=refnum<vi> refnum, vi path=w235, options=256) -> (vi reference=w251:refnum<vi>, error out=w250:errorcluster)  [unwired: 3 in]
        n121 = register-events(w239) -> ()  [unwired: 2 in, 2 out]
        n122 = call "supergui create stop queue.vi"() -> ("STOP Queue out"=w247:refnum<queue>)  [unwired: 11 in]
        n123 = Current VI's Menubar() -> (w240:refnum<k9>)
        n124 = call-by-ref "Start Asynchronous Call"(reference=w251, error in=w250, "STOP Queue in"=w247, "This Application"=w242, 8:"error in (no error)"=w245, "tcp data event"=w239, "Caller menu reference"=w240, "Caller VI ref"=w241) -> (reference out=w234:refnum<vi>, error out=w237:errorcluster)  [unwired: 5 in, 1 out]
        n125 = Bundle By Name(cluster=w244, "SuperGUI.SuperGUI ref"=w234, "SuperGUI.STOP queue"=w247) -> (w243:T24)
        n126 = call <vilib>:"Add State(s) to Queue__jki_lib_state_machine.vi"("State(s) in (\"\")"=w253) -> ("States Out"=w252:string)  [unwired: 14 in]
      }
      frame "UI: Stop SuperGUI" {
        # "Stop Supergui Clone and wait until it exit properly"
        n127 = Unbundle By Name(w256) -> ("SuperGUI.SuperGUI ref"=w258:refnum<vi>, "SuperGUI.STOP queue"=w257:refnum<queue>)
        n128 = Release Queue(queue=w257, error in (no error)=w255) -> (error out=w259:errorcluster)  [unwired: 1 in, 2 out]
        n129 = call-by-ref "Wait On Asynchronous Call"(reference=w258, error in=w259) -> ("error out"=w254:errorcluster)  [unwired: 11 in, 2 out]
        n130 = call <vilib>:"Add State(s) to Queue__jki_lib_state_machine.vi"("State(s) in (\"\")"=w261) -> ("States Out"=w260:string)  [unwired: 14 in]
      }
      frame "UI: Cursor Set" {
        # "Argument"
        # "Set and Unset Cursor Busy.\n(Usage: \"UI: Cursor Set >> Busy|Idle\")"
        n131 = case shown="\"Idle\", Default" w262 {
          tunnel: w264 -> [w269 w271]
          tunnel: [w268 w270] -> w263
          frame "Idle", Default {
            n132 = call <vilib>:"Unset Busy.vi"("error in (no error)"=w269) -> ("error out"=w268:errorcluster)  [unwired: 10 in]
          }
          frame "Busy" {
            n133 = call <vilib>:"Set Busy.vi"("error in (no error)"=w271) -> ("error out"=w270:errorcluster)  [unwired: 9 in, 1 out]
          }
        }
        n134 = call <vilib>:"Add State(s) to Queue__jki_lib_state_machine.vi"("State(s) in (\"\")"=w267) -> ("States Out"=w266:string)  [unwired: 14 in]
      }
      frame "UI: Front Panel State" {
        # "Argument"
        # "Set Front Panel Open or Closed\n(Usage: \"UI: Front Panel State >> Open|Close\")"
        n135 = Unbundle By Name(w274) -> ("Core.Current VI Reference"=w273:refnum<vi>)
        n136 = case shown="\"Open\", Default" w272 {
          tunnel: w276 -> [w282 w295]
          tunnel: [w284 w296] -> w275
          tunnel: w273 -> [w283 w293]
          frame "Open", Default {
            n137 = property class="VI"(reference=w283, error in=w282) -> (reference out=w280:refnum<vi>, error out=w281:errorcluster, "Front Panel.Open"=w279:bool)
            n138 = case shown="False" w279 {
              tunnel: [w287 w290] -> w284
              tunnel: w281 -> [w286 w290]
              tunnel: w280 -> [w285 _]
              frame False {
                n139 = invoke class="VI" method="FP.Open"(reference=w285, error in=w286, "Activate"=TRUE, "State"=T23."Standard") -> (error out=w287:errorcluster)  [unwired: 1 in, 4 out]
              }
              frame True {
              }
            }
          }
          frame "Close" {
            n140 = property class="VI"(reference=w293, error in=w295) -> (reference out=w292:refnum<vi>, error out=w294:errorcluster, "Front Panel.Open"=w291:bool)
            n141 = case shown="True" w291 {
              tunnel: [w297 w300] -> w296
              tunnel: w294 -> [w297 w299]
              tunnel: w292 -> [_ w298]
              frame False {
              }
              frame True {
                n142 = invoke class="VI" method="FP.Close"(reference=w298, error in=w299) -> (error out=w300:errorcluster)  [unwired: 1 in, 2 out]
              }
            }
          }
        }
        n143 = call <vilib>:"Add State(s) to Queue__jki_lib_state_machine.vi"("State(s) in (\"\")"=w278) -> ("States Out"=w277:string)  [unwired: 14 in]
      }
      frame "---------- Macro ----------" {
        # "Do not put any code in this frame.\n(It is a separator no-op. You can make a copy of this frame to create a new Macro frame)"
        n144 = call <vilib>:"Add State(s) to Queue__jki_lib_state_machine.vi"("State(s) in (\"\")"=w304) -> ("States Out"=w303:string)  [unwired: 14 in]
      }
      frame "Macro: Initialize" {
        # "Initialization Macro\n(This is called once, when the VI starts)"
        n145 = call <vilib>:"Add State(s) to Queue__jki_lib_state_machine.vi"("State(s) in Front (\"\")"="Data: Initialize\nInitialize Core Data\nUI: Initialize\nUI: Get Device Name\nUI: Start SuperGUI\nUI: Front Panel State >> Open", "State(s) in (\"\")"=w309) -> ("States Out"=w308:string)  [unwired: 13 in]
      }
      frame "Macro: Exit" {
        # "Exit Macro\n(This is called once, when the VI exits)"
        n146 = Unbundle By Name(w316) -> ("Core.Close Panel on Exit?"=w315:bool)
        n147 = Select(t="UI: Front Panel State >> Close", s=w315, f="") -> (s? t:f=w312:string)
        n148 = call <vilib>:"Add State(s) to Queue__jki_lib_state_machine.vi"("State(s) in (\"\")"=w312, "State(s) at Back (\"\")"="Data: Cleanup\nExit") -> ("States Out"=w310:string)  [unwired: 13 in]
        n149 = call <vilib>:"Add State(s) to Queue__jki_lib_state_machine.vi"("State(s) in Front (\"\")"=w310, "State(s) in (\"\")"=w319) -> ("States Out"=w318:string)  [unwired: 13 in]
      }
      frame "---------- New Category ----------" {
        # "Template Separator\n(You can make a copy of, or modify, this frame)"
        n150 = call <vilib>:"Add State(s) to Queue__jki_lib_state_machine.vi"("State(s) in (\"\")"=w323) -> ("States Out"=w322:string)  [unwired: 14 in]
      }
      frame "New Category: 1" {
        # "Your code here.\n(You can make a copy of, or modify, this frame)"
        n151 = call <vilib>:"Add State(s) to Queue__jki_lib_state_machine.vi"("State(s) in (\"\")"=w327) -> ("States Out"=w326:string)  [unwired: 14 in]
      }
      frame "New Category: 2" {
        # "Your code here.\n(You can make a copy of, or modify, this frame)"
        n152 = call <vilib>:"Add State(s) to Queue__jki_lib_state_machine.vi"("State(s) in (\"\")"=w331) -> ("States Out"=w330:string)  [unwired: 14 in]
      }
    }
    n153 = for {
      tunnel: w60 -> [w79]
      tunnel: w59 -> [w85]
      tunnel: w57 -> [w80] mode=indexing
      tunnel: w56 -> [w76]
      n154 = call-poly <userlib>:"Filter 1D Array__ogtk.vi"("items to filter"=w80, "array"=w85) -> ("filtered item indices"=w86:i32[])  [unwired: 4 in, 1 out]
      n155 = Index Array(array=w86) -> (element=w78:i32)  [unwired: 1 in]
      n156 = Index Array(array=w79, index=w78) -> (element=w84:T16)
      n157 = Index Array(array=w76, index=w78) -> (element=w77:T10)
      n158 = Unbundle By Name(w77) -> ("TargetSize.X::7"=w75:refnum<vi>, "TargetSize.Y::7"=w74:refnum<vi>)
      n159 = Unbundle By Name(w84) -> ("Target.X::7"=w88:refnum<vi>, "Target.Y::7"=w87:refnum<vi>)
      n160 = property class="DigNum (strict)"(reference=w88) -> ("Value"=w83:dbl)  [unwired: 1 in, 2 out]
      n161 = property class="DigNum (strict)"(reference=w87) -> ("Value"=w82:dbl)  [unwired: 1 in, 2 out]
      n162 = property class="DigNum (strict)"(reference=w75) -> ("Value"=w73:dbl)  [unwired: 1 in, 2 out]
      n163 = property class="DigNum (strict)"(reference=w74) -> ("Value"=w72:dbl)  [unwired: 1 in, 2 out]
      n164 = Bundle("Value"=w73, "Value"=w72) -> (w71:cluster{"Value":dbl, "Value":dbl})  [unwired: 1 in]
      n165 = call "draw crosshair imaq.vi"("Color"=u32 16774656, "Target.Y"=w82, "size"=w71, "Target.X"=w83, "Bounding Rectangle"=T20 {"Left"=0, "Top"=0, "Right"=0, "Bottom"=0}, "image in"=w80) -> ("error out"=→"error out":errorcluster)  [unwired: 4 in, 1 out]
    }
  }
